vi "Skipped.vi"(11 "Dummy In":refnum<class "Example Test Case.lvclass">) -> (0 "error out":errorcluster, 3 "Dummy Out":refnum<class "Example Test Case.lvclass">)   [LabVIEW 2020, in "Example Test Case.lvclass"]
doc: "Skipped test method"
uses:
  Example Test Case.lvclass
  C:/git/astemes-lunit/source/API/LUnit Test Case/LUnit Test Case.lvclass
  API/LUnit Test Case/LUnit Test Case.lvclass/LUnit Test Case.ctl
  API/LUnit Test Case/Private/Append Fail Result.vi
  API/LUnit Test Case/Private/Run In UI.vi
  <vilib>/Utility/error.llb/Clear Errors.vi
  Example Test Case.lvclass/Example Test Case.ctl
  API/LUnit Test Case/LUnit Test Case.lvclass
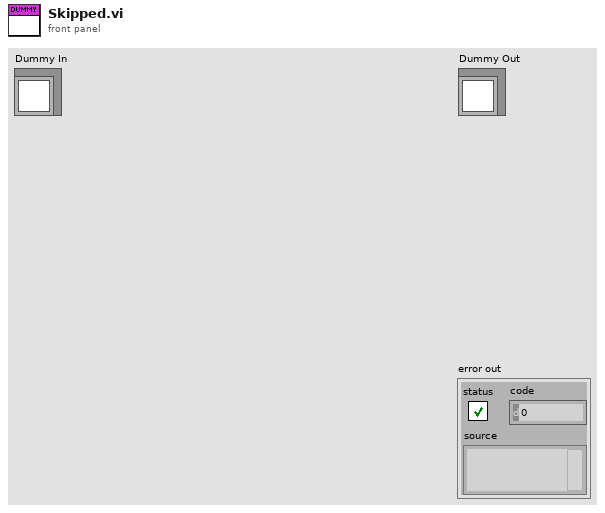
[diagram p1: front panel]
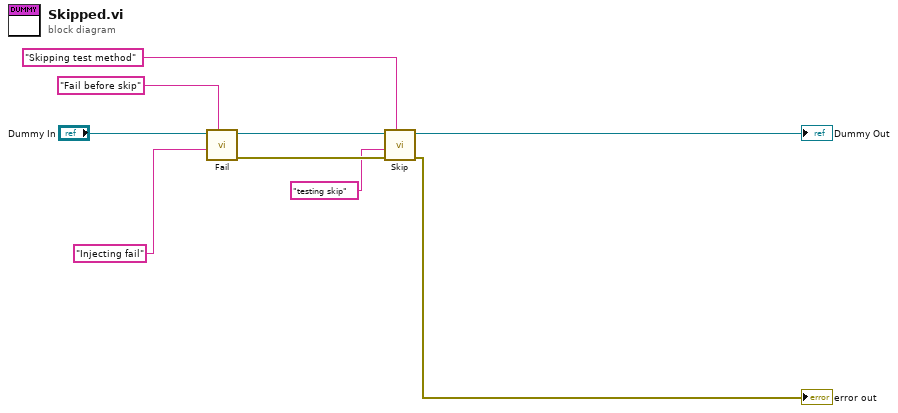
[diagram p0: block diagram]
diagram:
  n1 = call "Fail.vi"("Description"="Fail before skip", "Message"="Injecting fail", "LUnit Test Case In"="Dummy In") -> ("error out"=w5:errorcluster, "LUnit Test Case Out"=w6:refnum<class "Example Test Case.lvclass">)  [unwired: 7 in]
  n2 = call "Skip.vi"("Description"="Skipping test method", "error in (no error)"=w5, "Message"="testing skip", "LUnit Test Case In"=w6) -> ("error out"=→"error out":errorcluster, "LUnit Test Case Out"=→"Dummy Out":refnum<class "Example Test Case.lvclass">)  [unwired: 6 in]
